vi "Calc Eval.vi"(8 "error in (no error)":errorcluster, 10 "Inputs":dbl[](array[numeric]), 11 "Calculation in":refnum<class "Calculation.lvclass">) -> (0 "error out":errorcluster, 1 "Additional Updates":T1[](array[typedef]), 2 "Result":dbl, 3 "Calculation out":refnum<class "Calculation.lvclass">)   [LabVIEW 2020, in "VolatusCalcs.lvlib" / "Calculation.lvclass"]
uses:
  Calculation.lvclass
  Additional Update.ctl
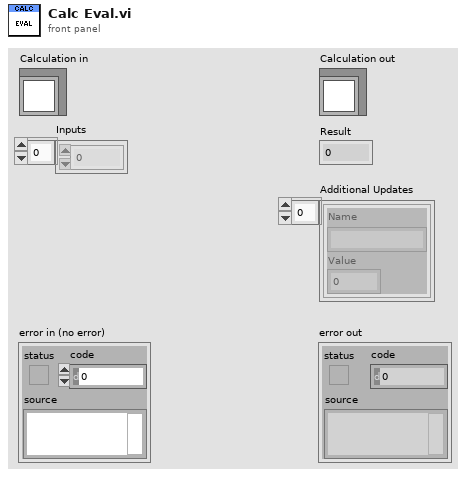
[diagram p1: front panel]
types:
  T1 = typedef "VolatusCalcs.lvlib/Calculation.lvclass/Additional Update.ctl" = cluster{"Name":string, "Value":dbl}
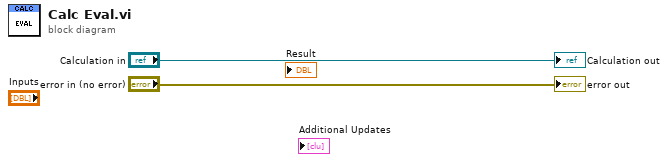
[diagram p0: block diagram]
diagram:
  "error out" <- "error in (no error)"
  "Calculation out" <- "Calculation in"
